vi "checkIfFilesExist.vi"(6 "Saved Tree":T1[](array[typedef]), 7 "Config Cluster out":T2, 8 "error in (no error)":errorcluster, 11 "Missing Files":refnum<vi>) -> (0 "error out":errorcluster, 1 "Files missing":bool, 2 "Missing Files":string[](array[string]))   [LabVIEW 2010]
uses:
  Config cluster.ctl
  ScriptStepTypeDef.ctl
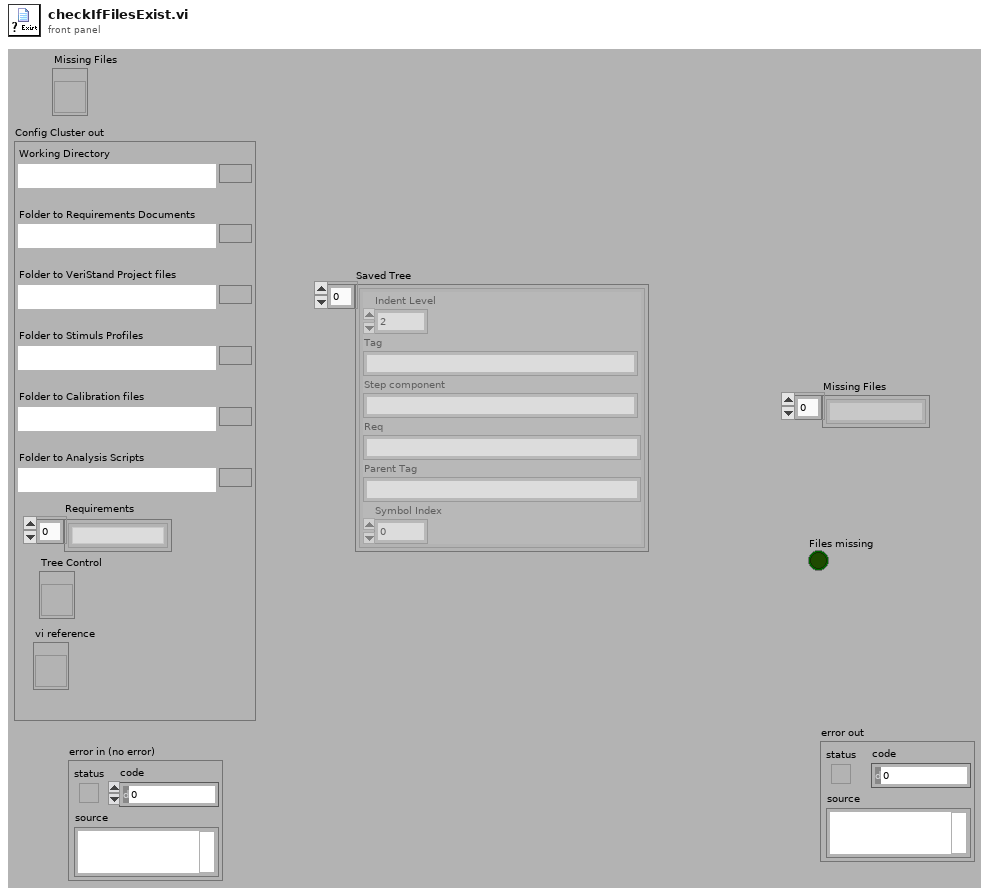
[diagram p1: front panel]
types:
  T1 = typedef "ScriptStepTypeDef.ctl" = cluster{"Indent Level":i32, "Tag":string, "Step component":string, "Req":string, "Parent Tag":string, "Symbol Index":i32}
  T2 = typedef "Config cluster.ctl" = cluster{"Working Directory":path, "Folder to Requirements Documents":path, "Folder to VeriStand Project files":path, "Folder to Stimuls Profiles":path, "Folder to Calibration files":path, "Folder to Analysis Scripts":path, "Requirements":string[], "Tree Control":refnum<vi>, "vi reference":refnum<vi>}
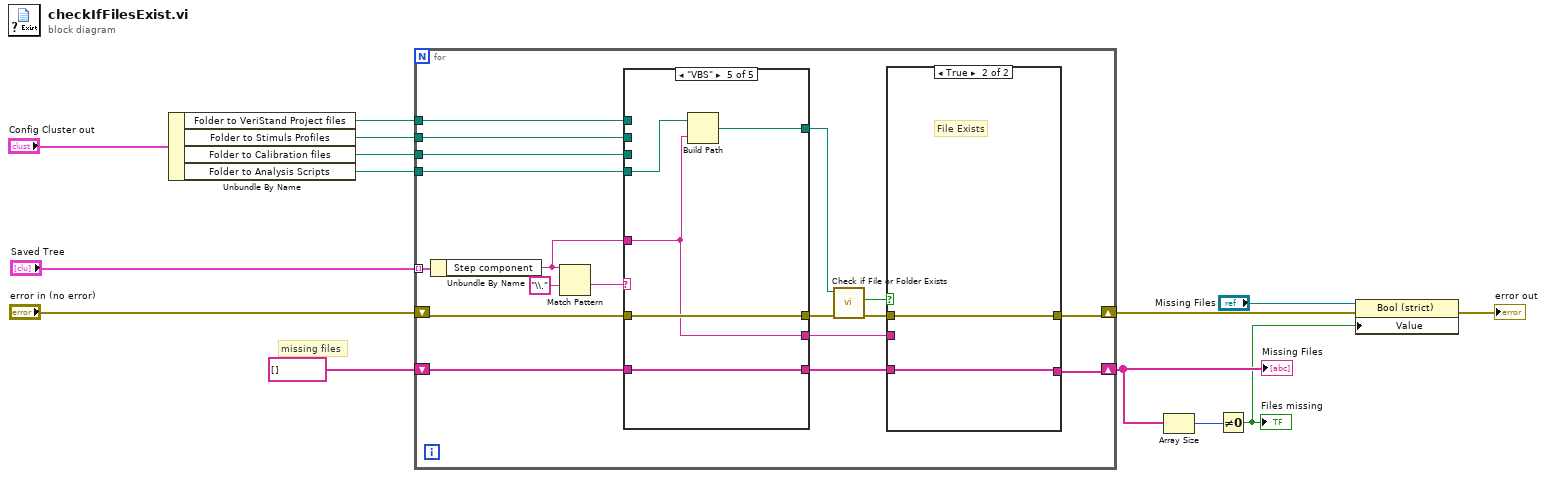
[diagram p0: block diagram]
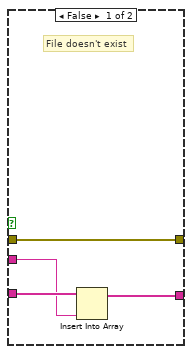
[diagram p2: hidden frame]
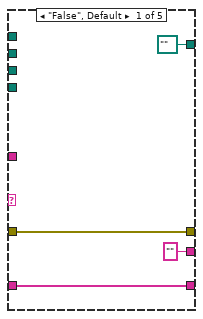
[diagram p3: hidden frame]
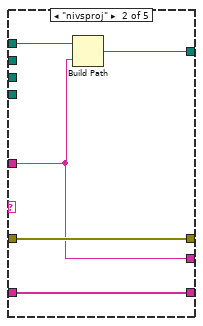
[diagram p4: hidden frame]
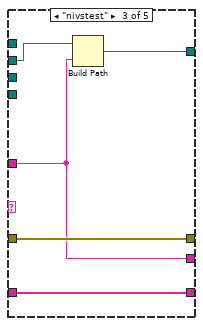
[diagram p5: hidden frame]
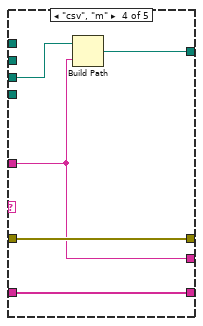
[diagram p6: hidden frame]
diagram:
  # "missing files"
  n1 = Unbundle By Name("Config Cluster out") -> ("Folder to VeriStand Project files"=w13:path, "Folder to Stimuls Profiles"=w12:path, "Folder to Calibration files"=w11:path, "Folder to Analysis Scripts"=w10:path)
  n2 = for {
    tunnel: w13 -> [w30]
    tunnel: w12 -> [w29]
    tunnel: w11 -> [w28]
    tunnel: w10 -> [w27]
    tunnel: "Saved Tree" -> [w32] mode=indexing
    shift-right: [w20] -> w3
    shift-left: "error in (no error)" -> [w25]
    shift-right: [w17] -> w5
    shift-left: string[] [] -> [w19]
    n3 = Unbundle By Name(w32) -> ("Step component"=w26:string)
    n4 = Match Pattern(string=w26, regular expression="\\.") -> (after substring=w16:string)  [unwired: 1 in, 3 out]
    n5 = case shown="\"VBS\"" w16 {
      tunnel: w30 -> [_ w47 _ _ _]
      tunnel: w29 -> [_ _ w49 _ _]
      tunnel: w28 -> [_ _ _ w54 _]
      tunnel: w27 -> [_ _ _ _ w59]
      tunnel: w26 -> [_ w43 w48 w53 w58]
      tunnel: w25 -> [w41 w46 w52 w57 w62]
      tunnel: [w41 w46 w52 w57 w62] -> w24
      tunnel: [path "" ("appended path") w45 w51 w56 w61] -> w23
      tunnel: w19 -> [w40 w44 w50 w55 w60]
      tunnel: [w40 w44 w50 w55 w60] -> w18
      tunnel: ["" ("Element name") w43 w48 w53 w58] -> w15
      frame "False", Default {
      }
      frame "nivsproj" {
        n6 = Build Path(base path=w47, name or relative path=w43) -> (appended path=w45:path)
      }
      frame "nivstest" {
        n7 = Build Path(base path=w49, name or relative path=w48) -> (appended path=w51:path)
      }
      frame "csv", "m" {
        n8 = Build Path(base path=w54, name or relative path=w53) -> (appended path=w56:path)
      }
      frame "VBS" {
        n9 = Build Path(base path=w59, name or relative path=w58) -> (appended path=w61:path)
      }
    }
    n10 = call <vilib>:"Check if File or Folder Exists.vi"("error in (no error)"=w24, "path"=w23) -> ("error out"=w21:errorcluster, "file or folder exists?"=w22:bool)  [unwired: 7 in, 1 out]
    n11 = case shown="True" w22 {
      tunnel: w21 -> [w36 w38]
      tunnel: [w36 w38] -> w20
      tunnel: w18 -> [w35 w37]
      tunnel: [w34 w37] -> w17
      tunnel: w15 -> [w33 _]
      frame False {
        # "File doesn't exist"
        n12 = Insert Into Array(array=w35, new element=w33) -> (w34:string[])  [unwired: 1 in]
      }
      frame True {
        # "File Exists"
      }
    }
  }
  "Missing Files" <- w5
  n13 = Array Size(array=w5) -> (size(s)=w6:i32)
  n14 = Not Equal To 0?(x=w6) -> (x != 0?=w1:bool)
  "Files missing" <- w1
  n15 = property class="Bool (strict)"(reference="Missing Files", error in=w3, "Value"=w1) -> (error out=→"error out":errorcluster)  [unwired: 1 out]
